vi "Camera Control.vi"() -> ()   [LabVIEW 2014]
uses:
  <vilib>/Platform/TimedLoop/XDataNode/timing_clust.ctl
  <vilib>/Platform/TimedLoop/XDataNode/nitl_modes.ctl
  <vilib>/Platform/TimedLoop/XDataNode/wakeup.ctl
  <vilib>/Platform/TimedLoop/XDataNode/XDataNode.xnode
  <vilib>/Platform/TimedLoop/XDataNode/XDNodeRunTimeDep.lvlib
panel:
  in  "Zoom Out 2":bool
  in  "Zoom In 2":bool
  in  "Zoom Out":bool
  in  "Zoom In":bool
  out "In use":bool
  in  "TCPConRef":refnum<k5>
  in  "Camera Down":bool
  in  "Camera Left":bool
  in  "Camera Right":bool
  in  "Camera Up":bool
  in  "CAMERA NO:":i8(knob) scale=1.0..4.0
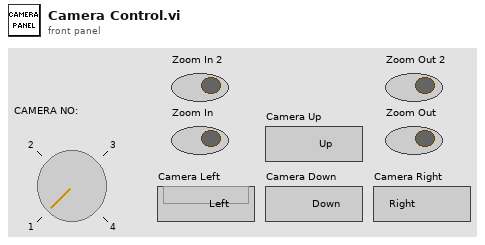
[diagram p1: front panel]
types:
  T1 = typedef "XDNodeRunTimeDep.lvlib/timing_clust.ctl" = cluster{"Expected End [f-1]":u64, "Actual End [f-1]":u64, "Finished Late? [f-1]":bool, "Expected End [i-1]":u64, "Actual End [i-1]":u64, "Finished Late? [i-1]":bool, "Expected Start [i]":u64, "Actual Start [i]":u64, "Expected Start [f]":u64, "Actual Start [f]":u64, "Source Name":string, "Structure Name":string, "Period":i64, "Deadline":i64, "Offset":i64, "Start":i64, "Priority":i32, "Timeout":i32, "Mode":T2, "Wakeup Reason":T3, "Error":errorcluster, "Source Type":string, "Secondary Source Type":string, "Global End Time":u64, "Global Start Time":u64, "Frame Duration":u64, "Iteration Duration":u64, "Assigned CPU":i32, "I/O Scan Engine Mode":u32}
  T2 = typedef "XDNodeRunTimeDep.lvlib/nitl_modes.ctl" = enum32{"No Change", "Process missed periods, maintain original phase", "Discard missed periods, maintain original phase", "Process missed periods, ignore original phase", "Discard missed periods, ignore original phase"}
  T3 = typedef "XDNodeRunTimeDep.lvlib/wakeup.ctl" = enum32{"Normal", "Aborted", "Asynchronous wakeup", "Timing source error", "Timed loop error", "Timeout"}
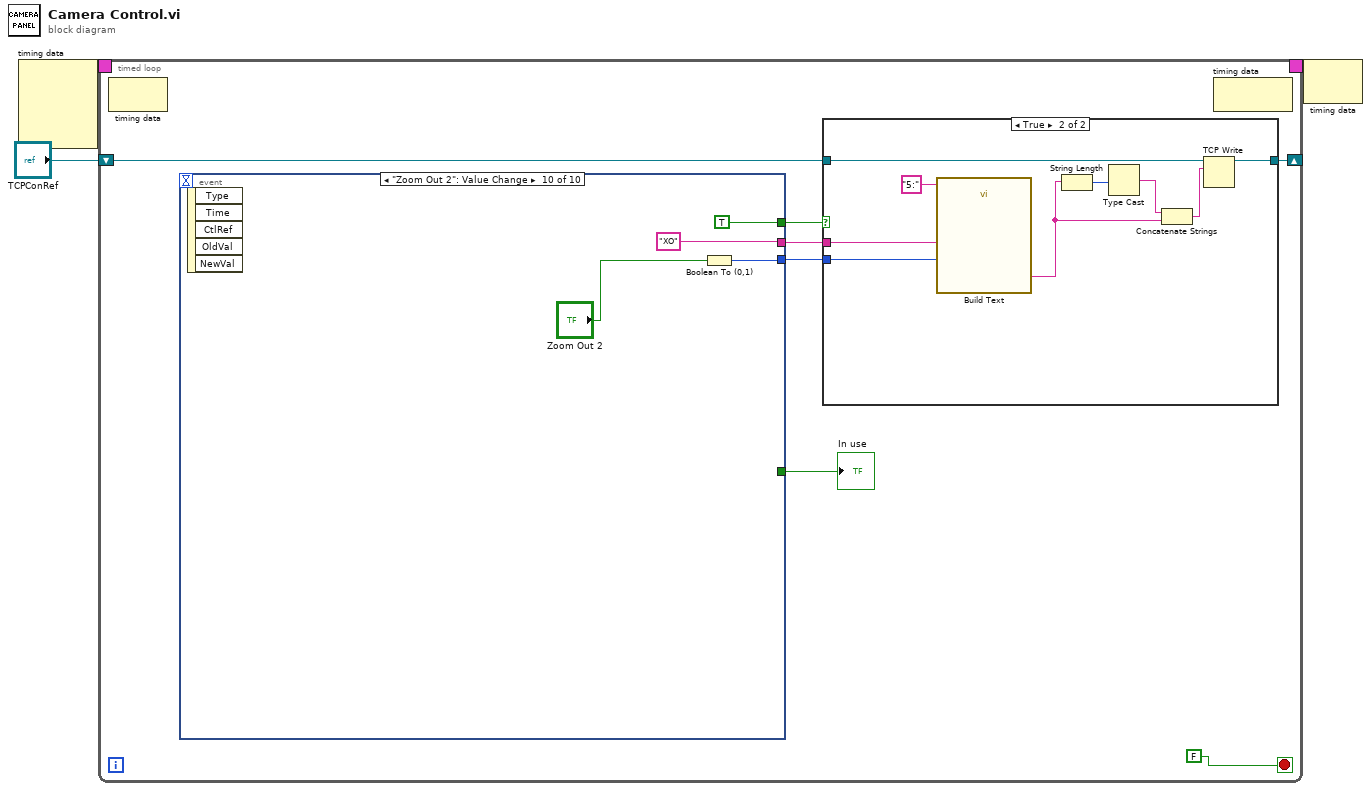
[diagram p0: block diagram]
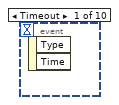
[diagram p3: hidden frame]
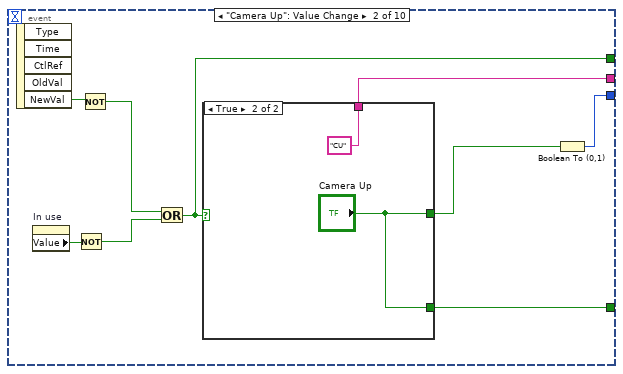
[diagram p4: hidden frame]
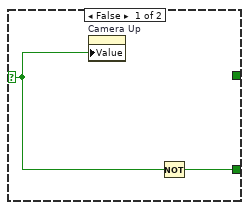
[diagram p5: hidden frame]
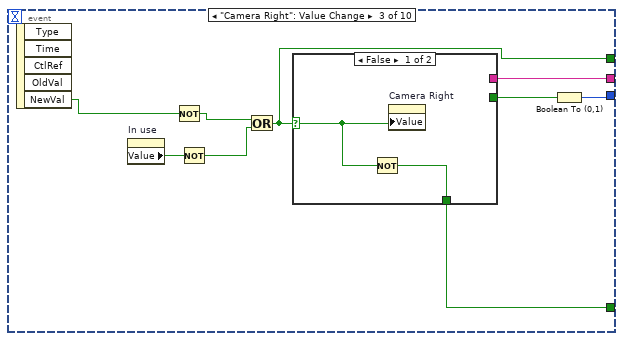
[diagram p6: hidden frame]
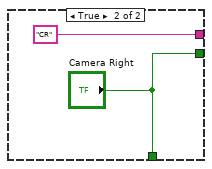
[diagram p7: hidden frame]
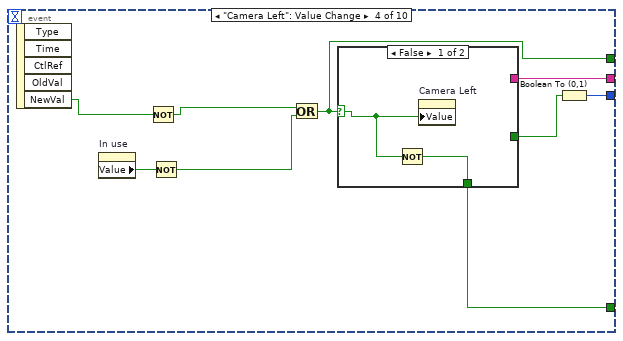
[diagram p8: hidden frame]
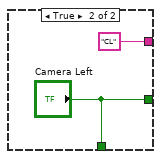
[diagram p9: hidden frame]
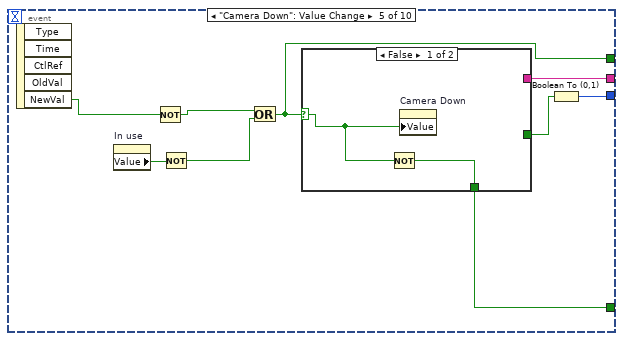
[diagram p10: hidden frame]
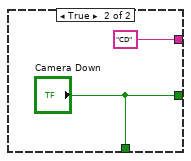
[diagram p11: hidden frame]
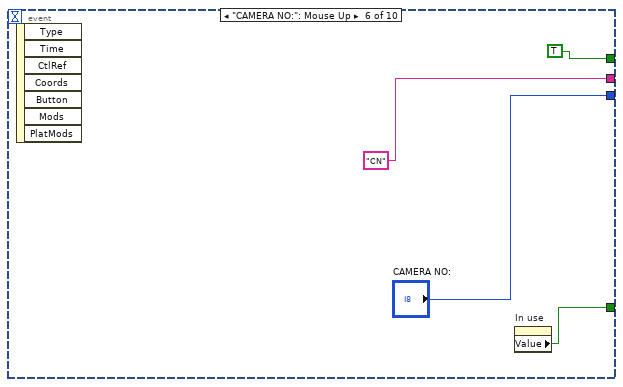
[diagram p12: hidden frame]
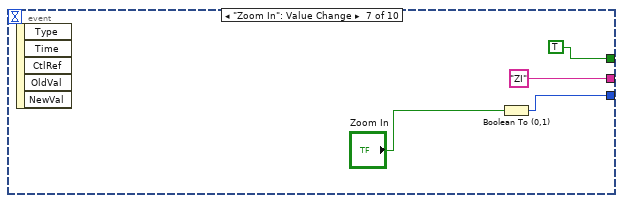
[diagram p13: hidden frame]
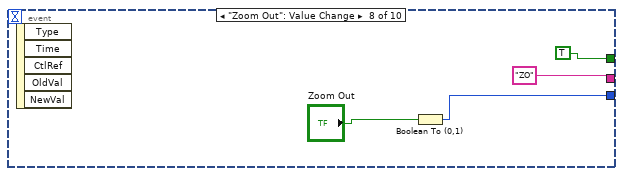
[diagram p14: hidden frame]
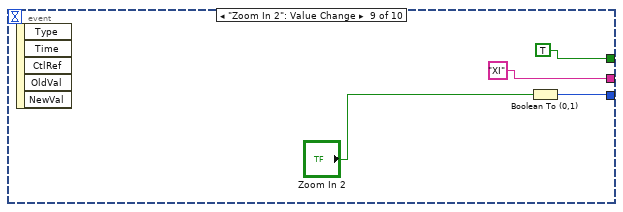
[diagram p15: hidden frame]
diagram:
  n1 = node-c288() -> (w2:T1)  [unwired: 4 in]
  n2 = timed-loop {
    shift-right: [w7] -> _
    shift-left: "TCPConRef" -> [w8]
    timing: w2 -> [_]
    timing-out: [_] -> w1
    stop <- FALSE stop-if-true
    n3 = node-c288() -> ()  [unwired: 1 in, 1 out]
    n4 = event shown="[9] \"Zoom Out 2\": Value Change" {
      selector: _ -> [_ _ _ _ _ _ _ _ _ _]
      dyn-events: _ -> [_ _ _ _ _ _ _ _ _ _]
      timeout: _ -> [_ _ _ _ _ _ _ _ _ _]
      tunnel: [_ w26 w44 w57 w70 "CN" "ZI" "ZO" "XI" "XO"] -> w10
      tunnel: [_ w31 w43 w56 w69 "CAMERA NO:" w81 w85 w89 w94] -> w9
      tunnel: [_ w24 w41 w54 w67 w76 _ _ _ _] -> w5
      tunnel: [_ w23 w36 w49 w62 TRUE TRUE TRUE TRUE TRUE] -> w4
      event Timeout {
        n5 = event-data() -> ()  [unwired: 1 in, 2 out]
      }
      event "Camera Up": Value Change {
        n6 = event-data() -> ("NewVal"=w29:bool)  [unwired: 1 in, 4 out]
        n7 = property on="In use" class="Bool (strict)"() -> ("Value"=w30:bool)  [unwired: 2 in, 2 out]
        n8 = Not(x=w30) -> (.not. x?=w28:bool)
        n9 = Not(x=w29) -> (.not. x?=w27:bool)
        n10 = Or(x=w27, y=w28) -> (x .or. y?=w23:bool)
        n11 = case shown="True" w23 {
          selector: w23 -> [w32 _]
          tunnel: [_ "CU"] -> w26
          tunnel: [_ "Camera Up"] -> w25
          tunnel: [w33 "Camera Up"] -> w24
          frame False {
            n12 = property on="Camera Up" class="Bool (strict)"("Value"=w32) -> ()  [unwired: 2 in, 2 out]
            n13 = Not(x=w32) -> (.not. x?=w33:bool)
          }
          frame True {
          }
        }
        n14 = Boolean To (0,1)(Boolean=w25) -> (0, 1=w31:i16)
      }
      event "Camera Right": Value Change {
        n15 = event-data() -> ("NewVal"=w37:bool)  [unwired: 1 in, 4 out]
        n16 = property on="In use" class="Bool (strict)"() -> ("Value"=w38:bool)  [unwired: 2 in, 2 out]
        n17 = Not(x=w37) -> (.not. x?=w40:bool)
        n18 = Not(x=w38) -> (.not. x?=w39:bool)
        n19 = Or(x=w40, y=w39) -> (x .or. y?=w36:bool)
        n20 = case shown="False" w36 {
          selector: w36 -> [w46 _]
          tunnel: [_ "CR"] -> w44
          tunnel: [_ "Camera Right"] -> w42
          tunnel: [w45 "Camera Right"] -> w41
          frame False {
            n21 = Not(x=w46) -> (.not. x?=w45:bool)
            n22 = property on="Camera Right" class="Bool (strict)"("Value"=w46) -> ()  [unwired: 2 in, 2 out]
          }
          frame True {
          }
        }
        n23 = Boolean To (0,1)(Boolean=w42) -> (0, 1=w43:i16)
      }
      event "Camera Left": Value Change {
        n24 = event-data() -> ("NewVal"=w52:bool)  [unwired: 1 in, 4 out]
        n25 = property on="In use" class="Bool (strict)"() -> ("Value"=w53:bool)  [unwired: 2 in, 2 out]
        n26 = Not(x=w52) -> (.not. x?=w51:bool)
        n27 = Not(x=w53) -> (.not. x?=w50:bool)
        n28 = Or(x=w51, y=w50) -> (x .or. y?=w49:bool)
        n29 = case shown="False" w49 {
          selector: w49 -> [w59 _]
          tunnel: [_ "CL"] -> w57
          tunnel: [_ "Camera Left"] -> w55
          tunnel: [w58 "Camera Left"] -> w54
          frame False {
            n30 = Not(x=w59) -> (.not. x?=w58:bool)
            n31 = property on="Camera Left" class="Bool (strict)"("Value"=w59) -> ()  [unwired: 2 in, 2 out]
          }
          frame True {
          }
        }
        n32 = Boolean To (0,1)(Boolean=w55) -> (0, 1=w56:i16)
      }
      event "Camera Down": Value Change {
        n33 = event-data() -> ("NewVal"=w64:bool)  [unwired: 1 in, 4 out]
        n34 = property on="In use" class="Bool (strict)"() -> ("Value"=w63:bool)  [unwired: 2 in, 2 out]
        n35 = Not(x=w64) -> (.not. x?=w66:bool)
        n36 = Not(x=w63) -> (.not. x?=w65:bool)
        n37 = Or(x=w66, y=w65) -> (x .or. y?=w62:bool)
        n38 = case shown="False" w62 {
          selector: w62 -> [w72 _]
          tunnel: [_ "CD"] -> w70
          tunnel: [_ "Camera Down"] -> w68
          tunnel: [w71 "Camera Down"] -> w67
          frame False {
            n39 = Not(x=w72) -> (.not. x?=w71:bool)
            n40 = property on="Camera Down" class="Bool (strict)"("Value"=w72) -> ()  [unwired: 2 in, 2 out]
          }
          frame True {
          }
        }
        n41 = Boolean To (0,1)(Boolean=w68) -> (0, 1=w69:i16)
      }
      event "CAMERA NO:": Mouse Up {
        n42 = event-data() -> ()  [unwired: 1 in, 7 out]
        n43 = property on="In use" class="Bool (strict)"() -> ("Value"=w76:bool)  [unwired: 2 in, 2 out]
      }
      event "Zoom In": Value Change {
        n44 = event-data() -> ()  [unwired: 1 in, 5 out]
        n45 = Boolean To (0,1)(Boolean="Zoom In") -> (0, 1=w81:i16)
      }
      event "Zoom Out": Value Change {
        n46 = event-data() -> ()  [unwired: 1 in, 5 out]
        n47 = Boolean To (0,1)(Boolean="Zoom Out") -> (0, 1=w85:i16)
      }
      event "Zoom In 2": Value Change {
        n48 = event-data() -> ()  [unwired: 1 in, 5 out]
        n49 = Boolean To (0,1)(Boolean="Zoom In 2") -> (0, 1=w89:i16)
      }
      event "Zoom Out 2": Value Change {
        n50 = event-data() -> ()  [unwired: 1 in, 5 out]
        n51 = Boolean To (0,1)(Boolean="Zoom Out 2") -> (0, 1=w94:i16)
      }
    }
    "In use" <- w5
    n52 = case shown="True" w4 {
      tunnel: w10 -> [_ w21]
      tunnel: w9 -> [_ w20]
      tunnel: w8 -> [w13 w19]
      tunnel: [w13 w18] -> w7
      frame False {
      }
      frame True {
        n53 = call "Build Text"("Beginning Text"="5:", "ControlID"=w21, "ControlValue"=w20) -> ("Result"=w15:string)  [unwired: 11 in, 1 out]
        n54 = String Length(string=w15) -> (length=w17:i32)
        n55 = Type Cast(x=w17) -> (*(type *) &x=w16:string)  [unwired: 1 in]
        n56 = Concatenate Strings(w16, w15) -> (w14:string)
        n57 = TCP Write(connection ID=w19, data in=w14) -> (connection ID out=w18:refnum<k5>)  [unwired: 2 in, 2 out]
      }
    }
    n58 = node-c288() -> ()  [unwired: 1 in, 1 out]
  }
  n59 = node-c288(w1) -> ()  [unwired: 1 out]
